vi "Write U32.vi"(8 "error in (no error)":errorcluster, 9 "offset (0)":u64 format="%d bytes", 10 "value":u32, 11 "Pointer in":refnum<class "Pointer.lvclass">) -> (0 "error out":errorcluster, 1 "offset + size":u64 format="%d bytes", 2 "value":u32, 3 "Pointer out":refnum<class "Pointer.lvclass">)   [LabVIEW 2020, in "Memory Manager.lvlib" / "Pointer.lvclass"]
doc: "Writes <b>value</b> to the address specified by <b>pointer + offset</b>."
uses:
  Pointer.lvclass
  Write (No Check) U32.vi
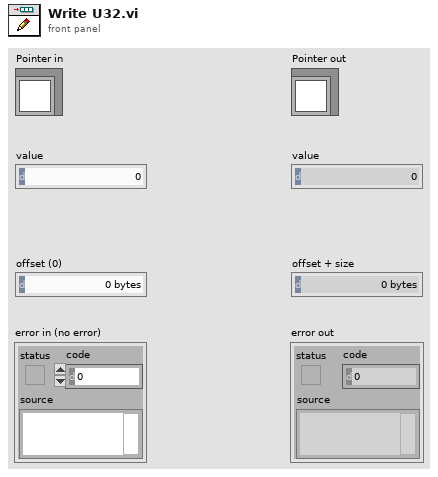
[diagram p1: front panel]
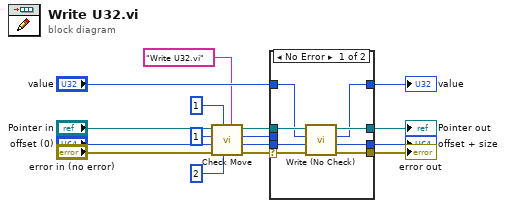
[diagram p0: block diagram]
diagram:
  n1 = call "Check Move.vi"("source vi name"="Write U32.vi", "count power of 2"=i16 2, "buffer count"=u64 1, "error in (no error)"="error in (no error)", "offset (0)"="offset (0)", "move count (-1: rest)"=i64 1, "Pointer in"="Pointer in") -> ("error out"=w15:errorcluster, "offset"=w14:u64, "count"=w13:u64, "Pointer out"=w16:refnum<class "Pointer.lvclass">)  [unwired: 1 in]
  n2 = case shown="No Error" w15 {
    selector: w15 -> [w24 w27]
    tunnel: w16 -> [w22 w26]
    tunnel: w14 -> [w23 w28]
    tunnel: "value" -> [w17 w25]
    tunnel: [w21 w27] -> w8
    tunnel: [w20 w26] -> w9
    tunnel: [w19 w28] -> w4
    tunnel: [w18 w25] -> w6
    tunnel: w13 -> [_ _]
    frame No Error {
      n3 = call-poly "Write (No Check).vi"("error in (no error)"=w24, "offset (0)"=w23, "value"=w17, "Pointer in"=w22) -> ("error out"=w21:errorcluster, "offset + size"=w19:u64, "value"=w18:u32, "Pointer out"=w20:refnum<class "Pointer.lvclass">)  [unwired: 4 in]
    }
    frame Error {
    }
  }
  "error out" <- w8
  "Pointer out" <- w9
  "value" <- w6
  "offset + size" <- w4
